vi "find_adapter_path.vi"(7 "source component path (if source not provided by object in)":path, 8 "error in (no error)":errorcluster, 10 "target component path":path, 11 "GenericComponent in":refnum<class "GenericComponent.lvclass">) -> (0 "error out":errorcluster, 2 "Path":path, 3 "GenericComponent out":refnum<class "GenericComponent.lvclass">)   [LabVIEW 2010, in "GenericComponent.lvclass"]
uses:
  GenericComponent.lvclass
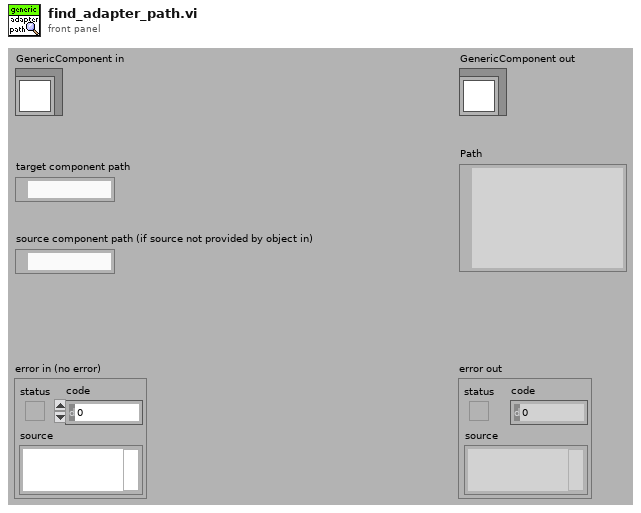
[diagram p1: front panel]
types:
  T1 = cluster{"substrings[0]":string, "substrings[1]":string, "substrings[2]":string}
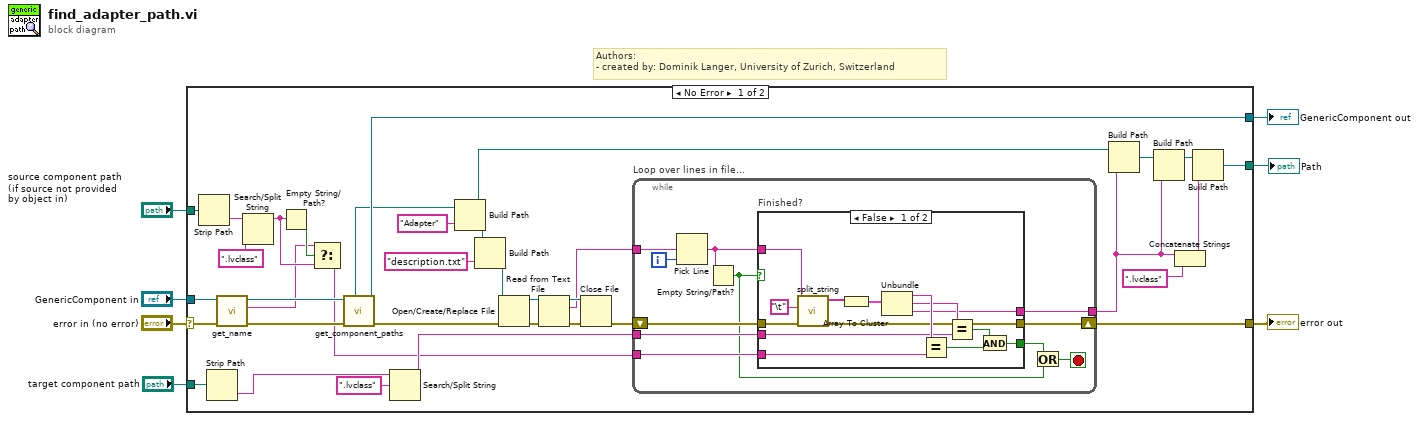
[diagram p0: block diagram]
diagram:
  # "Authors: \n- created by: Dominik Langer, University of Zurich, Switzerland"
  n1 = case shown="No Error" "error in (no error)" {
    selector: "error in (no error)" -> [w32 w70]
    tunnel: [w27 w70] -> w6
    tunnel: [w42 w69] -> w4
    tunnel: "GenericComponent in" -> [w30 w69]
    tunnel: "target component path" -> [w21 _]
    tunnel: [w23 _] -> w3
    tunnel: "source component path (if source not provided by object in)" -> [w14 _]
    frame No Error {
      n2 = Strip Path(path=w14) -> (name=w13:string)  [unwired: 1 out]
      n3 = Strip Path(path=w21) -> (name=w20:string)  [unwired: 1 out]
      n4 = call-dynamic "get_name.vi"("error in (no error)"=w32, "GenericPlugin in"=w30) -> ("error out"=w31:errorcluster, "component name"=w9:string, "GenericPlugin out"=w29:refnum<class "GenericComponent.lvclass">)  [unwired: 7 in]
      n5 = Search/Split String(string=w13, search string/char (-)=".lvclass") -> (substring before match=w10:string)  [unwired: 1 in, 2 out]
      n6 = Empty String/Path?(string/path=w10) -> (empty?=w11:bool)
      n7 = Select(t=w9, s=w11, f=w10) -> (s? t:f=w8:string)
      n8 = call-dynamic "get_component_paths.vi"("error in (no error)"=w31, "GenericComponent in"=w29) -> ("error out"=w22:errorcluster, "GenericComponent out"=w42:refnum<class "GenericComponent.lvclass">, "components directory"=w41:path)  [unwired: 4 in, 3 out]
      n9 = Search/Split String(string=w20, search string/char (-)=".lvclass") -> (substring before match=w18:string)  [unwired: 1 in, 2 out]
      n10 = Build Path(base path=w41, name or relative path="Adapter") -> (appended path=w26:path)
      n11 = Build Path(base path=w26, name or relative path="description.txt") -> (appended path=w36:path)
      n12 = Open/Create/Replace File(file path (use dialog)=w36, error in=w22) -> (refnum out=w35:refnum<file>, error out=w38:errorcluster)  [unwired: 4 in, 1 out]
      n13 = Read from Text File(file (use dialog)=w35, error in=w38) -> (refnum out=w34:refnum<file>, text=w33:string, error out=w37:errorcluster)  [unwired: 2 in, 1 out]
      n14 = Close File(refnum=w34, error in=w37) -> (error out=w28:errorcluster)  [unwired: 1 out]
      n15 = while "Loop over lines in file..." {
        tunnel: w33 -> [w52]
        tunnel: w8 -> [w50]
        tunnel: w18 -> [w48]
        shift-right: [w47] -> w27
        shift-left: w28 -> [w49]
        tunnel: [w43] -> w15
        i -> [w53]
        stop <- w44 stop-if-true
        n16 = Pick Line(multi-line string=w52, line index=w53) -> (output string=w51:string)  [unwired: 1 in]
        n17 = Empty String/Path?(string/path=w51) -> (empty?=w45:bool)
        n18 = case "Finished?" shown="False" w45 {
          tunnel: w51 -> [w66 _]
          tunnel: w50 -> [w62 _]
          tunnel: w49 -> [w67 w68]
          tunnel: w48 -> [w60 _]
          tunnel: [w58 w68] -> w47
          tunnel: [w55 _] -> w46
          tunnel: [w54 _] -> w43
          frame False {
            n19 = call "split_string.vi"("error in (no error)"=w67, "delimiter"="\t", "input string"=w66) -> ("error out"=w58:errorcluster, "substrings"=w64:string[])  [unwired: 7 in]
            n20 = Array To Cluster(array=w64) -> (cluster=w63:T1)
            n21 = Unbundle(w63) -> ("substrings[0]"=w61:string, "substrings[1]"=w59:string, "substrings[2]"=w54:string)
            n22 = Equal?(x=w61, y=w62) -> (x = y?=w56:bool)
            n23 = Equal?(x=w59, y=w60) -> (x = y?=w57:bool)
            n24 = And(x=w57, y=w56) -> (x .and. y?=w55:bool)
          }
          frame True {
          }
        }
        n25 = Or(x=w46, y=w45) -> (x .or. y?=w44:bool)
      }
      n26 = Build Path(base path=w26, name or relative path=w15) -> (appended path=w17:path)
      n27 = Build Path(base path=w17, name or relative path=w15) -> (appended path=w16:path)
      n28 = Concatenate Strings(w15, ".lvclass" ("string")) -> (w24:string)
      n29 = Build Path(base path=w16, name or relative path=w24) -> (appended path=w23:path)
    }
    frame Error {
    }
  }
  "error out" <- w6
  "GenericComponent out" <- w4
  "Path" <- w3
